vi "Server_Connection Check.vi"(8 "error in":errorcluster, 11 "Connection In":refnum<k5>) -> (0 "error out":errorcluster, 2 "Disconnected":bool, 3 "Connection out":refnum<k5>)   [LabVIEW 2018, in "Cloud Server.lvlib"]
uses:
  Cloud Server.lvlib
  Data Def/Server_Connection Manager Method.ctl
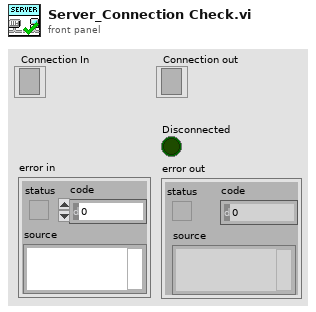
[diagram p1: front panel]
types:
  T1 = typedef "Cloud Server.lvlib/Server_Connection Manager Method.ctl" = enum16{"Initialize", "Add", "Get", "Set Properties", "Get Properties", "Close", "Release"}
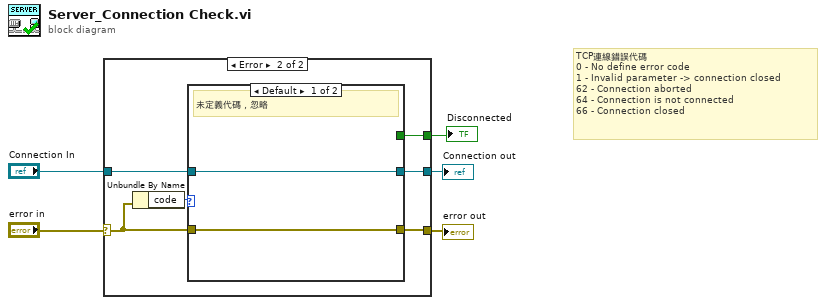
[diagram p0: block diagram]
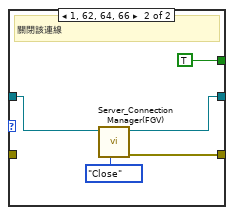
[diagram p3: hidden frame]
diagram:
  # "TCP連線錯誤代碼\n0 - No define error code\n1 - Invalid parameter -> connection closed\n62 - Connection aborted\n64 - Connection is not connected\n66 - Connection closed"
  n1 = case shown="Error" "error in" {
    selector: "error in" -> [w7 w12]
    tunnel: [w7 w11] -> w4
    tunnel: "Connection In" -> [w6 w10]
    tunnel: [w6 w9] -> w2
    tunnel: [_ w8] -> w1
    frame No Error {
    }
    frame Error {
      n2 = Unbundle By Name(w12) -> ("code"=w13:i32)
      n3 = case shown="Default" w13 {
        tunnel: w12 -> [w15 _]
        tunnel: [w15 w19] -> w11
        tunnel: w10 -> [w14 w18]
        tunnel: [w14 w17] -> w9
        tunnel: [_ TRUE] -> w8
        frame Default {
          # "未定義代碼，忽略"
        }
        frame 1, 62, 64, 66 {
          # "關閉該連線"
          n4 = call "Server_Connection Manager(FGV).vi"("Connection Manager Method(Get)"=Server_Connection_Manager_Method."Close", "Connection In"=w18) -> ("error out"=w19:errorcluster, "Connection Out"=w17:refnum<k5>)  [unwired: 5 in, 3 out]
        }
      }
    }
  }
  "error out" <- w4
  "Connection out" <- w2
  "Disconnected" <- w1
